vi "rectangular_sample_setup.vi"(9 "A (mm)":dbl, 10 "B (mm)":dbl, 11 "L (mm)":dbl) -> (1 "Result":dbl, 3 "spreadsheet string":string)   [LabVIEW 2011]
uses:
  <vilib>/express/express arith-compare/Formula/XNode/ExpressFormulaBlockNode.xnode
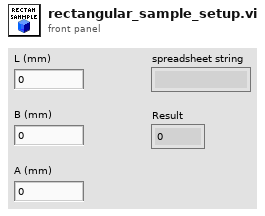
[diagram p1: front panel]
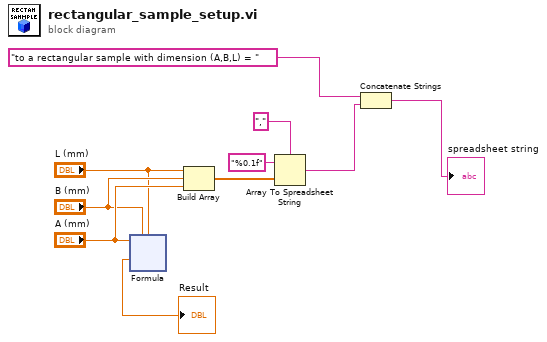
[diagram p0: block diagram]
diagram:
  n1 = xnode "Formula"("A"="A (mm)", "B"="B (mm)", "L"="L (mm)") -> ("Result"=→"Result":dbl)  [unwired: 1 in, 1 out]
  n2 = Build Array("L (mm)", "B (mm)", "A (mm)") -> (w3:dbl[])
  n3 = Array To Spreadsheet String(delimiter (Tab)=",", array=w3, 3:"%0.1f" ("format string")) -> (spreadsheet string=w10:string)
  n4 = Concatenate Strings("to a rectangular sample with dimension (A,B,L) = " ("string"), w10) -> (→"spreadsheet string":string)
